vi "Clarke (FXP).vi"(2 "B":fxp<+/-,32,5>, 3 "A":fxp<+/-,32,5>) -> (0 "beta":fxp<+/-,32,5> format="%.30g", 1 "alpha":fxp<+/-,32,5> format="%.29g")   [LabVIEW 2025]
uses:
  <vilib>/rvi/FXPMathLib/FxpMul/XNode/nifxpmath_Multiplier.xnode
  <vilib>/rvi/FXPMathLib/sim/FxpSim.dll
  <vilib>/rvi/FXPMathLib/FxpAdd/XNode/nifxpmath_Add.xnode
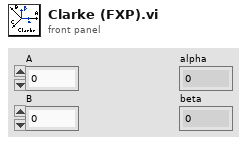
[diagram p1: front panel]
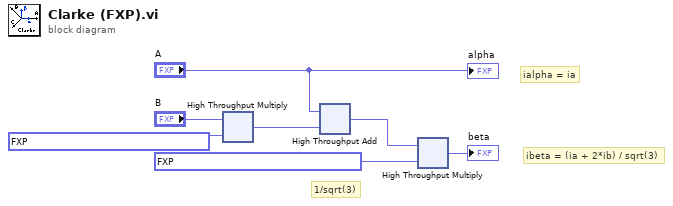
[diagram p0: block diagram]
diagram:
  # "ibeta = (ia + 2*ib) / sqrt(3)"
  # "ialpha = ia"
  # "1/sqrt(3)"
  n1 = xnode "High Throughput Multiply"("x"="B", "y"=fxp<+,32,1> 1.9999999995343387) -> ("x*y"=w7:fxp<+/-,32,6>)
  n2 = xnode "High Throughput Add"("x"="A", "y"=w7) -> ("x+y"=w2:fxp<+/-,32,6>)
  n3 = xnode "High Throughput Multiply"("x"=w2, "y"=fxp<+,32,0> 0.5773502693045884) -> ("x*y"=→"beta":fxp<+/-,32,5>)
  "alpha" <- "A"
